vi "Release Tree Manager.vi"(8 "Error In":errorcluster, 11 "Tree":refnum<data-value>) -> (0 "Error Out":errorcluster)   [LabVIEW 2017, in "Tree API.lvlib" / "Tree.lvclass"]
doc: "Releases an obtained reference to the Tree Manager. Tries to invoke the safe Release method on all Tree Data attributes."
uses:
  Tree.lvclass
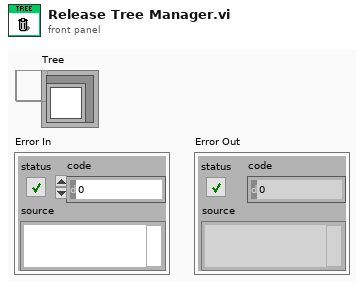
[diagram p1: front panel]
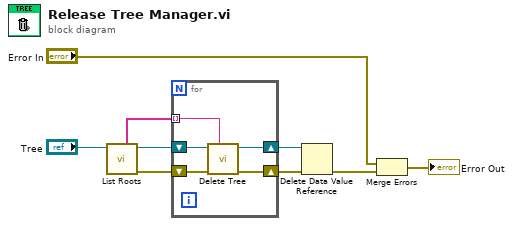
[diagram p0: block diagram]
diagram:
  n1 = call "List Roots.vi"("Tree"="Tree") -> ("Error Out"=w4:errorcluster, "Tree"=w5:refnum<data-value>, "Roots IDs"=w6:string[])  [unwired: 7 in, 1 out]
  n2 = for {
    tunnel: w6 -> [w14] mode=indexing
    shift-right: [w11] -> w3
    shift-left: w5 -> [w13]
    shift-right: [w10] -> w2
    shift-left: w4 -> [w12]
    n3 = call "Delete Tree.vi"("Tree ID"=w14, "Error In"=w12, "Tree Manager"=w13) -> ("Error Out"=w10:errorcluster, "Tree Manager"=w11:refnum<data-value>)  [unwired: 7 in]
  }
  n4 = Delete Data Value Reference(data value reference=w3, error in=w2) -> (error out=w1:errorcluster)  [unwired: 1 out]
  n5 = Merge Errors("Error In", w1) -> (→"Error Out":errorcluster)
